vi "Display_Temp.vi"() -> ()   [LabVIEW 2024]
uses:
  <vilib>/Utility/file.llb/Write Delimited Spreadsheet (DBL).vi
panel:
  out "T > Soglia":u32
  out "Allarme":bool
  in  "Soglia °C":dbl=38.0
  in  "file path (dialog if empty)":path
  in  "STOP":bool
  out "Gradi Centrigradi OUT":dbl
  out "Waveform Chart":T1(graph)
  out "Temp (F)":dbl(slide) scale=0.0..110.0
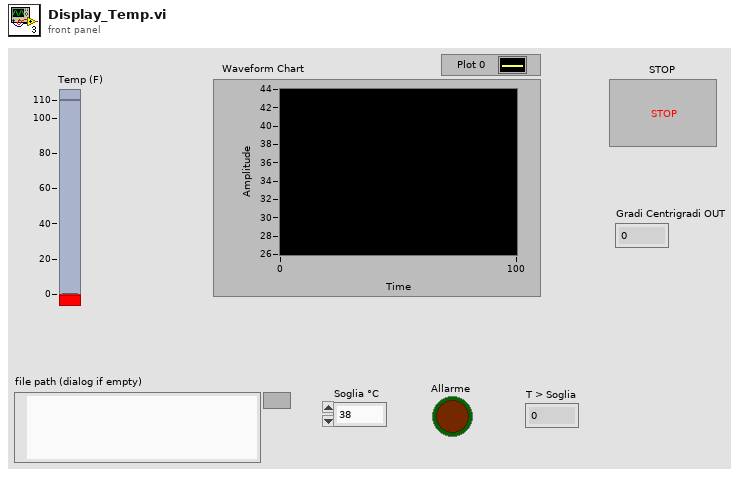
[diagram p1: front panel]
types:
  T1 = cluster{"Gradi Centrigradi OUT":dbl, "Soglia °C":dbl}
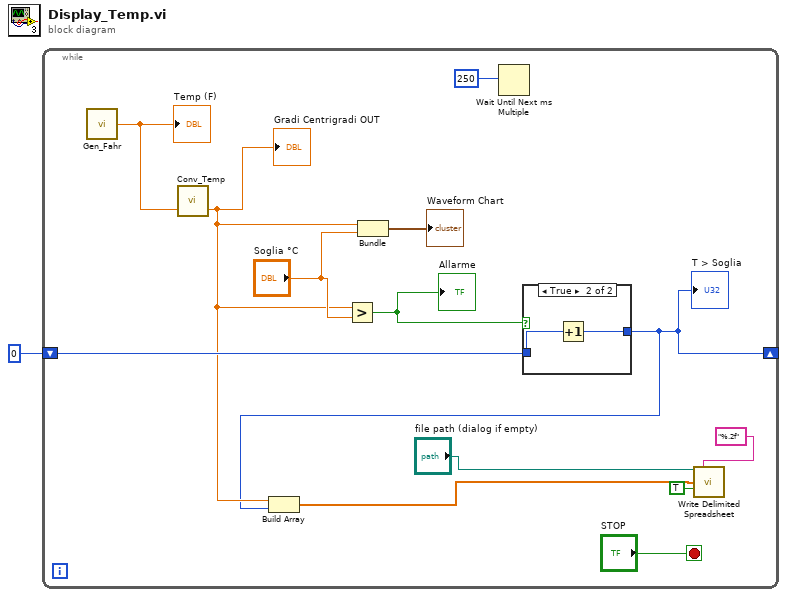
[diagram p0: block diagram]
diagram:
  n1 = while {
    shift-right: [w3] -> _
    shift-left: u32 0 -> [w8]
    stop <- "STOP" stop-if-true
    n2 = call "Gen_Fahr.vi"() -> ("Temp (F)"=w14:dbl)  [unwired: 1 in]
    "Temp (F)" <- w14
    n3 = call "Conv_Temp.vi"("Gradi Fahrenheit IN"=w14) -> ("Gradi Centrigradi OUT"=w4:dbl)  [unwired: 1 in, 1 out]
    "Gradi Centrigradi OUT" <- w4
    n4 = Greater?(x=w4, y="Soglia °C") -> (0:w9:bool)
    "Allarme" <- w9
    n5 = Bundle("Gradi Centrigradi OUT"=w4, "Soglia °C"="Soglia °C") -> (→"Waveform Chart":T1)  [unwired: 1 in]
    n6 = Wait Until Next ms Multiple(millisecond multiple=250) -> ()  [unwired: 1 out]
    n7 = case shown="True" w9 {
      tunnel: w8 -> [w15 w17]
      tunnel: [w15 w16] -> w3
      frame False {
      }
      frame True {
        n8 = Increment(x=w17) -> (x+1=w16:u32)
      }
    }
    "T > Soglia" <- w3
    n9 = Build Array(w4, w3) -> (w2:dbl[])
    n10 = call-poly <vilib>:"Write Delimited Spreadsheet.vi"("file path (dialog if empty)"="file path (dialog if empty)", "format (%.3f)"="%.2f", "1D data"=w2, "append to file? (new file:F)"=TRUE) -> ()  [unwired: 10 in, 2 out]
  }
